vi "color_selector.vi"(10 "state":bool) -> (2 "Colors [4]":cluster{u32, u32}[](array[cluster]))   [LabVIEW 2015]
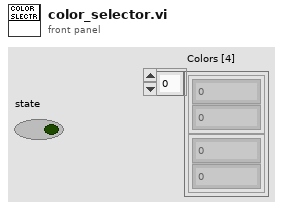
[diagram p1: front panel]
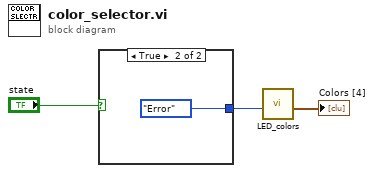
[diagram p0: block diagram]
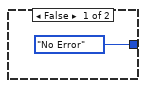
[diagram p2: hidden frame]
diagram:
  n1 = case shown="True" "state" {
    tunnel: [enum16{"Default", "Error", "No Error"}."No Error" ("state") enum16{"Default", "Error", "No Error"}."Error" ("state")] -> w3
    frame False {
    }
    frame True {
    }
  }
  n2 = call "LED_colors.vi"("state"=w3) -> ("Colors [4]"=→"Colors [4]":cluster{u32, u32}[])  [unwired: 10 in]
